vi "Scans at different Bias.vi"() -> ()   [LabVIEW 2021]
doc: "This example performs multiple image scans, increasing the bias voltage after each scan.\n\n- Nanonis Programming Interface -"
uses:
  Nanonis Prog Interface.lvlib
panel:
  in  "Auto save":bool
  in  "Serie name":string="ScanMultiBias_"
  in  "Bias increment":sgl=0.1
  out "Scan":u8 caption="Current scan"
  in  "Number of scans":u8=5
  out "Bias voltage":sgl caption="Current bias voltage"
  # "Example program for the Nanonis SPM Control software programming interface\n(see diagram)."
  # "This example performs multiple image scans, increasing the bias voltage after each scan."
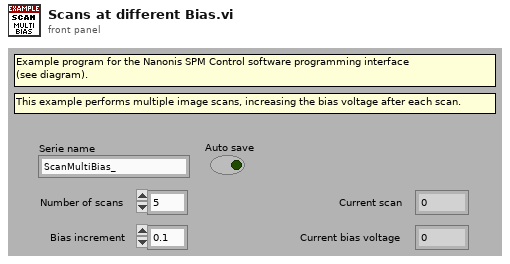
[diagram p1: front panel]
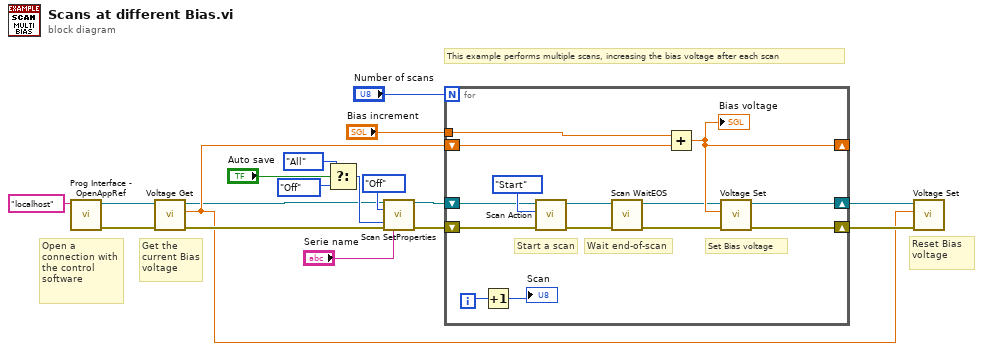
[diagram p0: block diagram]
diagram:
  # "Reset Bias voltage"
  # "Open a connection with the control\nsoftware"
  # "This example performs multiple scans, increasing the bias voltage after each scan"
  # "Get the current Bias voltage"
  n1 = call <userlib>:"Prog Interface - OpenAppRef.vi"("Machine name (local machine IP)"="localhost" ("Machine name (localhost)")) -> ("Error out"=w16:errorcluster, "Application reference"=w4:refnum<vi>)  [unwired: 5 in]
  n2 = call <userlib>:"Voltage Get.vi"("error in (no error)"=w16, "Application ref in"=w4) -> ("error out"=w14:errorcluster, "Bias (V)"=w10:sgl, "Application ref out"=w3:refnum<vi>)  [unwired: 7 in]
  n3 = Select(t=enum16{"No change", "All", "Next", "Off"}."All" ("Auto save"), s="Auto save", f=enum16{"No change", "All", "Next", "Off"}."Off" ("Auto save")) -> (s? t:f=w5:enum16{"No change", "All", "Next", "Off"})
  n4 = call <userlib>:"Scan SetProperties.vi"("Application ref in"=w3, "Continuous scan"=enum16{"No change", "On", "Off"}."Off", "Auto save"=w5, "Error in (no error)"=w14, "Serie name"="Serie name") -> ("Application ref out"=w2:refnum<vi>, "Error out"=w13:errorcluster)  [unwired: 9 in]
  n5 = for {
    N: "Number of scans" -> [_]
    tunnel: "Bias increment" -> [w32]
    shift-right: [w31] -> w11
    shift-left: w13 -> [w28]
    shift-right: [w24] -> _
    shift-left: w10 -> [w25]
    shift-right: [w19] -> w1
    shift-left: w2 -> [w22]
    i -> [w30]
    # "Set Bias voltage"
    # "Wait end-of-scan"
    # "Start a scan"
    n6 = Increment(x=w30) -> (x+1=→"Scan":i32)
    n7 = call <userlib>:"Scan Action.vi"("error in (no error)"=w28, "Scan action (Start)"=enum16{"Start", "Stop", "Pause", "Resume"}."Start" ("Scan action"), "Application ref in"=w22) -> ("error out"=w27:errorcluster, "Application ref out"=w21:refnum<vi>)  [unwired: 6 in]
    n8 = call <userlib>:"Scan WaitEOS.vi"("error in (no error)"=w27, "Application ref in"=w21) -> ("error out"=w26:errorcluster, "Application ref out"=w20:refnum<vi>)  [unwired: 5 in, 2 out]
    n9 = Add(x=w32, y=w25) -> (x+y=w24:sgl)
    "Bias voltage" <- w24
    n10 = call <userlib>:"Voltage Set.vi"("Error in (no error)"=w26, "Bias (V)"=w24, "Application ref in"=w20) -> ("Error out"=w31:errorcluster, "Application ref out"=w19:refnum<vi>)  [unwired: 7 in]
  }
  n11 = call <userlib>:"Voltage Set.vi"("Error in (no error)"=w11, "Bias (V)"=w10, "Application ref in"=w1) -> ()  [unwired: 7 in, 2 out]
